vi "Arrays 1.vi"() -> ()   [LabVIEW 2014]
panel:
  out "Subset":dbl[](array[numeric])
  out "min index":i32
  out "max index":i32
  out "min value":dbl
  out "max value":dbl
  out "size":i32
  in  "Stop Button":bool
  in  "Array":dbl[](array[numeric])
  # "Arrays - First VI"
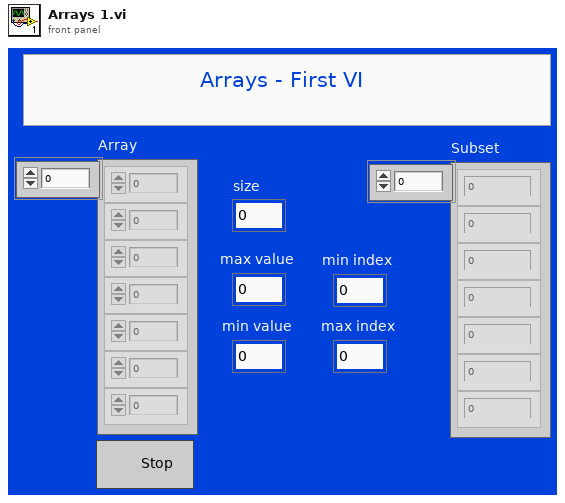
[diagram p1: front panel]
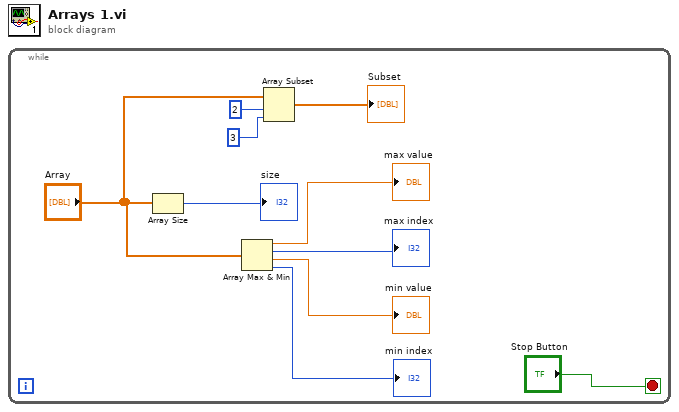
[diagram p0: block diagram]
diagram:
  n1 = while {
    stop <- "Stop Button" stop-if-true
    n2 = Array Size(array="Array") -> (size(s)=→"size":i32)
    n3 = Array Max & Min(array="Array") -> (max value=→"max value":dbl, max index (indices)=→"max index":i32, min value=→"min value":dbl, min index (indices)=→"min index":i32)
    n4 = Array Subset(array="Array", index=2, length=3) -> (→"Subset":dbl[])
  }
